vi "Update SquareBattle Project.vi"() -> ()   [LabVIEW 2020]
uses:
  dev/Version.ctl
  dev/Updater State.ctl
  fab92dee-f5cc-474f-8dc6-a01214f8643b.vi
  <vilib>/Comparison/Equal/Equal Functor/Equal Functor.lvclass
panel:
  out "Project":refnum<vi>
  out "Template Vers Str":string
  out "Project Vers Str":string
  out "Template Version":T1
  out "Project Version":T1
  out "Template Project":path
  out "Progress":u16(slide) scale=0.0..100.0
  out "Status":string
  out "Squares":path[](array[path])
  out "App Folder":path
  out "Engine Folder":path
  out "Project Path":path
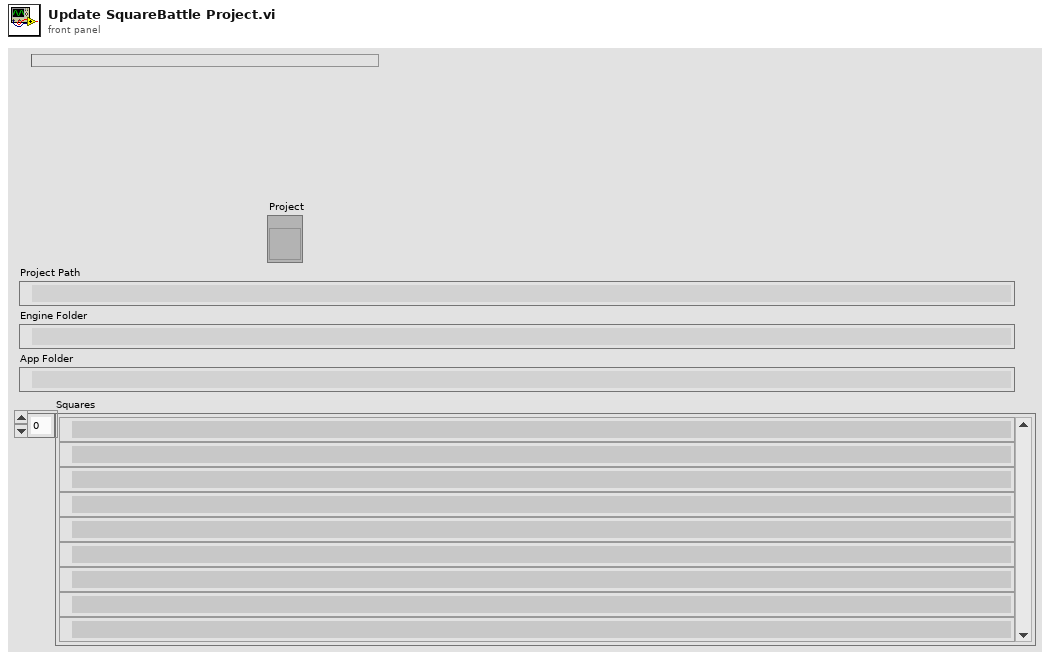
[diagram p1: front panel]
types:
  T1 = typedef "Version.ctl" = cluster{"Major":u16, "Minor":u16, "Fix":u16, "Build":u16}
  T2 = typedef "Updater State.ctl" = enum16{"Get References", "Check Versions", "Confirm", "Close Project", "Copy Engine", "Copy Squares", "Open Project", "Version Scripting", "Close"}
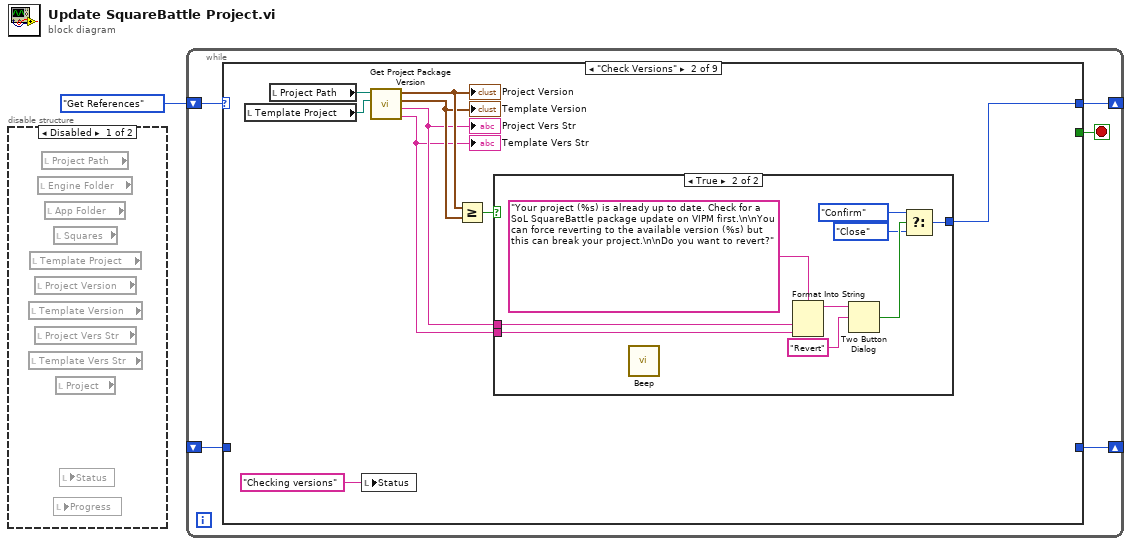
[diagram p0: block diagram]
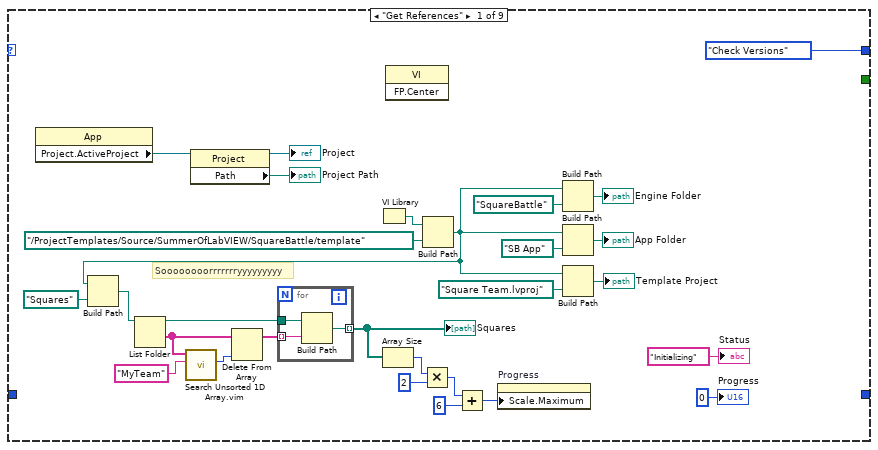
[diagram p3: hidden frame]
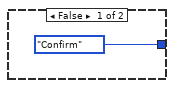
[diagram p4: hidden frame]
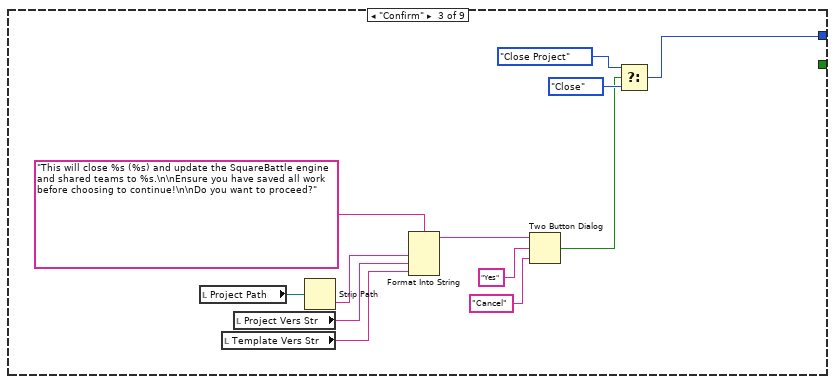
[diagram p5: hidden frame]
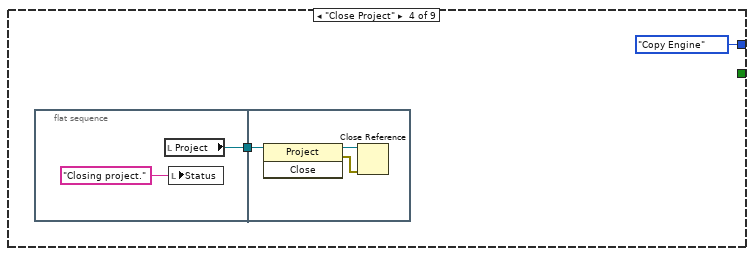
[diagram p6: hidden frame]
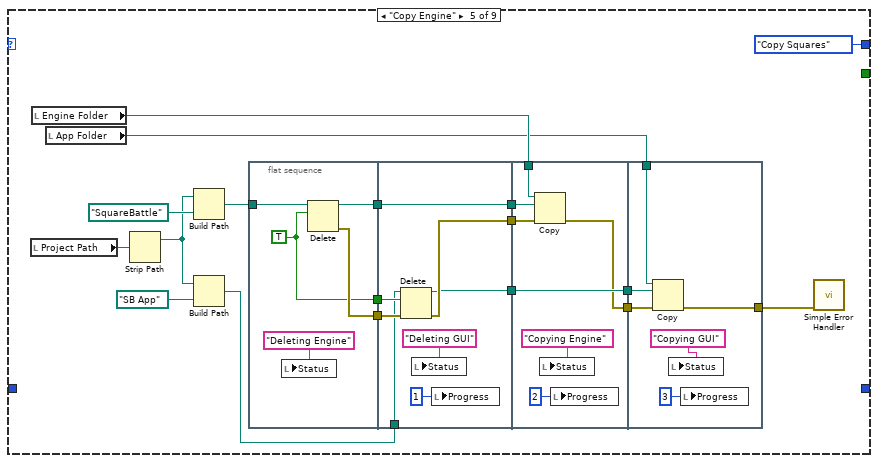
[diagram p7: hidden frame]
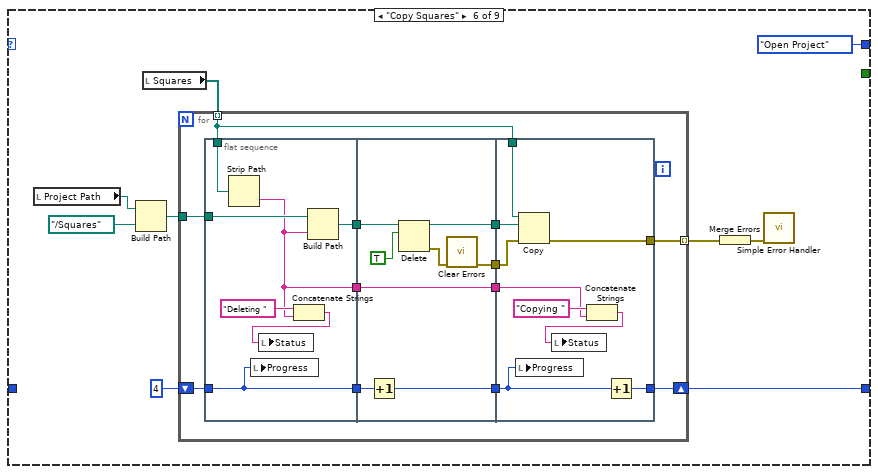
[diagram p8: hidden frame]
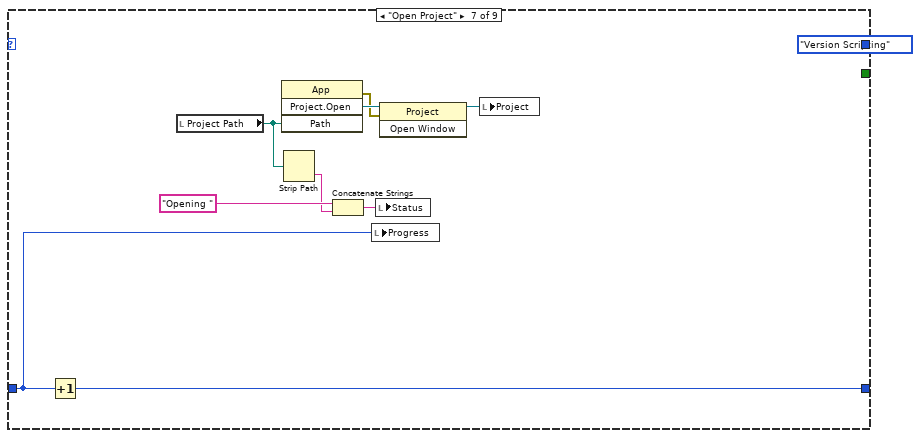
[diagram p9: hidden frame]
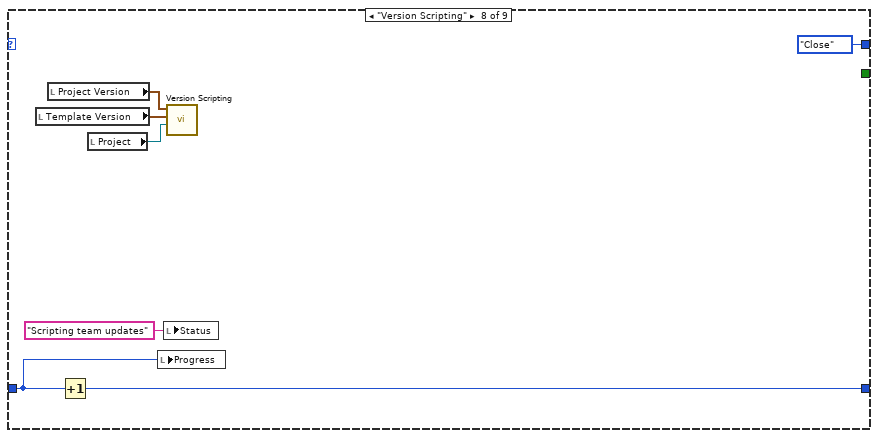
[diagram p10: hidden frame]
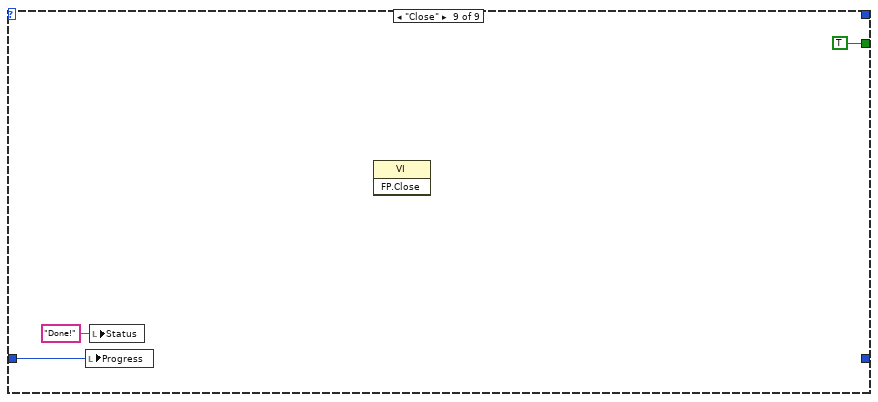
[diagram p11: hidden frame]
diagram:
  n1 = disable-structure shown="Disabled" {
    frame Disabled {
      n2 = local read "Template Version"() -> ()  [unwired: 1 out]
      n3 = local read "Template Vers Str"() -> ()  [unwired: 1 out]
      n4 = local read "Template Project"() -> ()  [unwired: 1 out]
      n5 = local read "Project Version"() -> ()  [unwired: 1 out]
      n6 = local read "Project Vers Str"() -> ()  [unwired: 1 out]
      n7 = local read "Engine Folder"() -> ()  [unwired: 1 out]
      n8 = local read "Project Path"() -> ()  [unwired: 1 out]
      n9 = local read "App Folder"() -> ()  [unwired: 1 out]
      n10 = local read "Squares"() -> ()  [unwired: 1 out]
      n11 = local read "Progress"() -> ()  [unwired: 1 in]
      n12 = local read "Project"() -> ()  [unwired: 1 out]
      n13 = local read "Status"() -> ()  [unwired: 1 in]
    }
    frame Enabled {
    }
  }
  n14 = while {
    shift-right: [w5] -> _
    shift-left: Updater_State."Get References" -> [w6]
    shift-right: [w3] -> _
    shift-left: _ -> [w2]
    stop <- w4 stop-if-true
    n15 = case shown="\"Check Versions\"" w6 {
      tunnel: [Updater_State."Check Versions" ("f") w40 w63 Updater_State."Copy Engine" ("f") Updater_State."Copy Squares" ("f") Updater_State."Open Project" ("f") Updater_State."Version Scripting" ("f") Updater_State."Close" ("f") _] -> w5
      tunnel: [_ _ _ _ _ _ _ _ TRUE] -> w4
      tunnel: [_ _ _ _ _ w120 w166 w175 _] -> w3
      tunnel: w2 -> [_ _ _ _ _ _ w167 w176 w183]
      frame "Get References" {
        # "Soooooooorrrrrrryyyyyyyyy"
        n16 = property class="App"() -> ("Project.ActiveProject"=w10:refnum<vi>)  [unwired: 2 in, 2 out]
        n17 = property class="Project"(reference=w10) -> (reference out=→"Project":refnum<vi>, "Path"=→"Project Path":path)  [unwired: 1 in, 1 out]
        n18 = VI Library() -> (path=w32:path)
        n19 = invoke class="VI" method="FP.Center"() -> ()  [unwired: 3 in, 3 out]
        n20 = Build Path(base path=w32, name or relative path=path "../ProjectTemplates/Source/SummerOfLabVIEW/SquareBattle/template") -> (appended path=w9:path)
        n21 = Build Path(base path=w9, name or relative path=path "Squares") -> (appended path=w25:path)
        n22 = List Folder(path=w25) -> (path out=w20:path, folder names=w23:string[])  [unwired: 3 in, 2 out]
        n23 = call "Search Unsorted 1D Array.vim"("element"="MyTeam", "unsorted 1D array"=w23) -> ("index of element"=w22:i32)  [unwired: 9 in]
        n24 = Delete From Array(array=w23, index=w22) -> (array with subset deleted=w21:string[])  [unwired: 1 in, 1 out]
        n25 = for {
          tunnel: w21 -> [w36] mode=indexing
          tunnel: w20 -> [w37]
          tunnel: [w35] -> w18 mode=indexing
          n26 = Build Path(base path=w37, name or relative path=w36) -> (appended path=w35:path)
        }
        "Squares" <- w18
        n27 = Array Size(array=w18) -> (size(s)=w17:i32)
        n28 = Multiply(x=w17, y=2) -> (x*y=w15:i32)
        n29 = Add(x=w15, y=6) -> (x+y=w13:i32)
        n30 = property on="Progress" class="Slide (strict)"("Scale.Maximum"=w13) -> ()  [unwired: 2 in, 2 out]
        n31 = Build Path(base path=w9, name or relative path=path "SquareBattle") -> (appended path=→"Engine Folder":path)
        n32 = Build Path(base path=w9, name or relative path=path "SB App") -> (appended path=→"App Folder":path)
        n33 = Build Path(base path=w9, name or relative path=path "Square Team.lvproj") -> (appended path=→"Template Project":path)
        "Status" <- "Initializing" ("Status")
        "Progress" <- u16 0 ("Progress")
      }
      frame "Check Versions" {
        n34 = local read "Template Project"() -> (w44:path)
        n35 = local read "Project Path"() -> (w46:path)
        n36 = local write "Status"("Checking versions" ("Status")) -> ()
        n37 = call "Get Project Package Version.vi"("Template Project"=w44, "Project Path"=w46) -> ("Template Vers Str"=w38:string, "Project Vers Str"=w39:string, "Template Version"=w42:T1, "Project Version"=w43:T1)  [unwired: 6 in]
        "Project Version" <- w43
        "Template Version" <- w42
        "Project Vers Str" <- w39
        "Template Vers Str" <- w38
        n38 = Greater Or Equal?(x=w43, y=w42) -> (x >= y?=w41:bool)
        n39 = case shown="True" w41 {
          tunnel: [Updater_State."Confirm" ("f") w48] -> w40
          tunnel: w39 -> [_ w55]
          tunnel: w38 -> [_ w54]
          frame False {
          }
          frame True {
            n40 = call <vilib>:"Beep.vi"() -> ()  [unwired: 12 in]
            n41 = Format Into String(format string="Your project (%s) is already up to date. Check for a SoL SquareBattle package update on VIPM first.\n\nYou can force reverting to the available version (%s) but this can break your project.\n\nDo you want to revert?" ("message"), w55, w54) -> (resulting string=w53:string)  [unwired: 2 in, 1 out]
            n42 = Two Button Dialog(message=w53, 2:"Revert" ("T button name (\"OK\")")) -> (T button?=w51:bool)  [unwired: 1 in]
            n43 = Select(t=Updater_State."Confirm" ("f"), s=w51, f=Updater_State."Close") -> (s? t:f=w48:T2)
          }
        }
      }
      frame "Confirm" {
        n44 = local read "Project Path"() -> (w61:path)
        n45 = local read "Template Vers Str"() -> (w57:string)
        n46 = local read "Project Vers Str"() -> (w58:string)
        n47 = Strip Path(path=w61) -> (name=w60:string)  [unwired: 1 out]
        n48 = Format Into String(format string="This will close %s (%s) and update the SquareBattle engine and shared teams to %s.\n\nEnsure you have saved all work before choosing to continue!\n\nDo you want to proceed?" ("message"), w60, w58, w57) -> (resulting string=w59:string)  [unwired: 2 in, 1 out]
        n49 = Two Button Dialog(message=w59, 1:"Cancel" ("F button name (\"Cancel\")"), 2:"Yes" ("T button name (\"OK\")")) -> (T button?=w64:bool)
        n50 = Select(t=Updater_State."Close Project", s=w64, f=Updater_State."Close") -> (s? t:f=w63:T2)
      }
      frame "Close Project" {
        n51 = flat-sequence {
          tunnel: [w71] -> w69
          tunnel: w69 -> [w73]
          frame #0 {
            n52 = local read "Project"() -> (w71:refnum<vi>)
            n53 = local write "Status"("Closing project." ("Status")) -> ()
          }
          frame #1 {
            n54 = invoke class="Project" method="Close"(reference=w73) -> (reference out=w75:refnum<vi>, error out=w74:errorcluster)  [unwired: 2 in, 1 out]
            n55 = Close Reference(reference=w75, error in (no error)=w74) -> ()  [unwired: 1 out]
          }
        }
      }
      frame "Copy Engine" {
        n56 = local read "Project Path"() -> (w93:path)
        n57 = local read "Engine Folder"() -> (w80:path)
        n58 = local read "App Folder"() -> (w77:path)
        n59 = Strip Path(path=w93) -> (stripped path=w90:path)  [unwired: 1 out]
        n60 = Build Path(base path=w90, name or relative path=path "SquareBattle") -> (appended path=w89:path)
        n61 = Build Path(base path=w90, name or relative path=path "SB App") -> (appended path=w84:path)
        n62 = flat-sequence {
          tunnel: w89 -> [w97]
          tunnel: [w98] -> w87
          tunnel: [w96] -> w86
          tunnel: [w95] -> w85
          tunnel: w87 -> [w105]
          tunnel: w86 -> [w106]
          tunnel: w85 -> [w104]
          tunnel: w84 -> [w103]
          tunnel: [w106] -> w83
          tunnel: [w102] -> w82
          tunnel: [w101] -> w81
          tunnel: w83 -> [w111]
          tunnel: w82 -> [w112]
          tunnel: w81 -> [w113]
          tunnel: w80 -> [w110]
          tunnel: [w113] -> w79
          tunnel: [w109] -> w78
          tunnel: w79 -> [w118]
          tunnel: w78 -> [w119]
          tunnel: w77 -> [w117]
          tunnel: [w116] -> w76
          frame #0 {
            w95 = TRUE ("entire hierarchy (F)")
            n63 = local write "Status"("Deleting Engine") -> ()
            n64 = Delete(path (use dialog)=w97, entire hierarchy (F)=w95) -> (deleted path=w96:path, error out=w98:errorcluster)  [unwired: 3 in, 1 out]
          }
          frame #1 {
            n65 = Delete(path (use dialog)=w103, entire hierarchy (F)=w104, error in=w105) -> (deleted path=w101:path, error out=w102:errorcluster)  [unwired: 2 in, 1 out]
            n66 = local write "Status"("Deleting GUI") -> ()
            n67 = local write "Progress"(u16 1 ("Progress")) -> ()
          }
          frame #2 {
            n68 = Copy(8:w112, 10:w111, 11:w110) -> (0:w109:errorcluster)  [unwired: 2 in, 2 out]
            n69 = local write "Status"("Copying Engine") -> ()
            n70 = local write "Progress"(u16 2 ("Progress")) -> ()
          }
          frame #3 {
            n71 = Copy(8:w119, 10:w118, 11:w117) -> (0:w116:errorcluster)  [unwired: 2 in, 2 out]
            n72 = local write "Status"("Copying GUI") -> ()
            n73 = local write "Progress"(u16 3 ("Progress")) -> ()
          }
        }
        n74 = call <vilib>:"Simple Error Handler.vi"("error in (no error)"=w76) -> ()  [unwired: 4 in, 5 out]
      }
      frame "Copy Squares" {
        n75 = local read "Project Path"() -> (w128:path)
        n76 = Build Path(base path=w128, name or relative path=path "../Squares") -> (appended path=w125:path)
        n77 = local read "Squares"() -> (w126:path[])
        n78 = for {
          tunnel: w126 -> [w136] mode=indexing
          tunnel: w125 -> [w140]
          tunnel: [w135] -> w124 mode=indexing
          shift-right: [w129] -> w120
          shift-left: u16 4 ("Progress") -> [w132]
          n79 = flat-sequence {
            tunnel: w140 -> [w147]
            tunnel: w136 -> [w145]
            tunnel: [w146] -> w139
            tunnel: [w142] -> w133
            tunnel: w132 -> [w141]
            tunnel: [w141] -> w131
            tunnel: w139 -> [w153]
            tunnel: [w152] -> w138
            tunnel: [w151] -> w137
            tunnel: [w150] -> w134
            tunnel: w133 -> [w150]
            tunnel: w131 -> [w149]
            tunnel: [w148] -> w130
            tunnel: w138 -> [w164]
            tunnel: w137 -> [w163]
            tunnel: w136 -> [w162]
            tunnel: [w161] -> w135
            tunnel: w134 -> [w156]
            tunnel: w130 -> [w160]
            tunnel: [w159] -> w129
            frame #0 {
              n80 = Strip Path(path=w145) -> (name=w142:string)  [unwired: 1 out]
              n81 = local write "Progress"(w141) -> ()
              n82 = Concatenate Strings("Deleting ", w142) -> (w143:string)
              n83 = local write "Status"(w143) -> ()
              n84 = Build Path(base path=w147, name or relative path=w142) -> (appended path=w146:path)
            }
            frame #1 {
              n85 = Increment(x=w149) -> (x+1=w148:u16)
              n86 = Delete(path (use dialog)=w153, entire hierarchy (F)=TRUE) -> (deleted path=w151:path, error out=w155:errorcluster)  [unwired: 3 in, 1 out]
              n87 = call <vilib>:"Clear Errors.vi"("error in (no error)"=w155) -> ("error out"=w152:errorcluster)  [unwired: 5 in, 1 out]
            }
            frame #2 {
              n88 = local write "Progress"(w160) -> ()
              n89 = Copy(8:w164, 10:w163, 11:w162) -> (0:w161:errorcluster)  [unwired: 2 in, 2 out]
              n90 = Concatenate Strings("Copying ", w156) -> (w158:string)
              n91 = local write "Status"(w158) -> ()
              n92 = Increment(x=w160) -> (x+1=w159:u16)
            }
          }
        }
        n93 = Merge Errors(w124) -> (w123:errorcluster)
        n94 = call <vilib>:"Simple Error Handler.vi"("error in (no error)"=w123) -> ()  [unwired: 4 in, 5 out]
      }
      frame "Open Project" {
        n95 = Increment(x=w167) -> (x+1=w166:u16)
        n96 = local read "Project Path"() -> (w171:path)
        n97 = invoke class="App" method="Project.Open"("Path"=w171) -> (error out=w172:errorcluster, "Project:Open"=w173:refnum<vi>)  [unwired: 3 in, 2 out]
        n98 = Strip Path(path=w171) -> (name=w169:string)  [unwired: 1 out]
        n99 = Concatenate Strings("Opening " ("Status"), w169) -> (w168:string)
        n100 = local write "Progress"(w167) -> ()
        n101 = local write "Status"(w168) -> ()
        n102 = invoke class="Project" method="Open Window"(reference=w173, error in=w172) -> (reference out=w165:refnum<vi>)  [unwired: 1 in, 2 out]
        n103 = local write "Project"(w165) -> ()
      }
      frame "Version Scripting" {
        n104 = local read "Template Version"() -> (w181:T1)
        n105 = local read "Project Version"() -> (w180:T1)
        n106 = Increment(x=w176) -> (x+1=w175:u16)
        n107 = local read "Project"() -> (w179:refnum<vi>)
        n108 = local write "Progress"(w176) -> ()
        n109 = local write "Status"("Scripting team updates" ("Status")) -> ()
        n110 = call "Version Scripting.vi"("Project"=w179, "To"=w181, "From"=w180) -> ()  [unwired: 9 in]
      }
      frame "Close" {
        n111 = local write "Progress"(w183) -> ()
        n112 = local write "Status"("Done!" ("Status")) -> ()
        n113 = invoke class="VI" method="FP.Close"() -> ()  [unwired: 3 in, 3 out]
      }
    }
  }
